vi "埃德1.vi"() -> ()   [LabVIEW 2017]
uses:
  <vilib>/vision/Pattern Matching.llb/IMAQ GM Match Report.ctl
panel:
  out "Matches (Geometric Matching 1)":T1[](array[typedef]) {"Correlation Score" format="%.2f"; "Target Template Curve Score" format="%.2f"; "Template Target Curve Score" format="%.2f"; "Bounding Box"."y" format="%.2f"; "Bounding Box"."x" format="%.2f"; "Position"."y" format="%.2f"; "Position"."x" format="%.2f"; "Score" format="%.2f"; "Scale" format="%.2f"; "Angle" format="%.2f"; "Occlusion %" format="%.2f"}
  out "路径":path
  out "数值":i32
  in  "毫秒计时值":u32
  out "Image":T2(plugin-control)
  out "All Files in Dir":path[](array[path]) caption="目录中的所有文件"
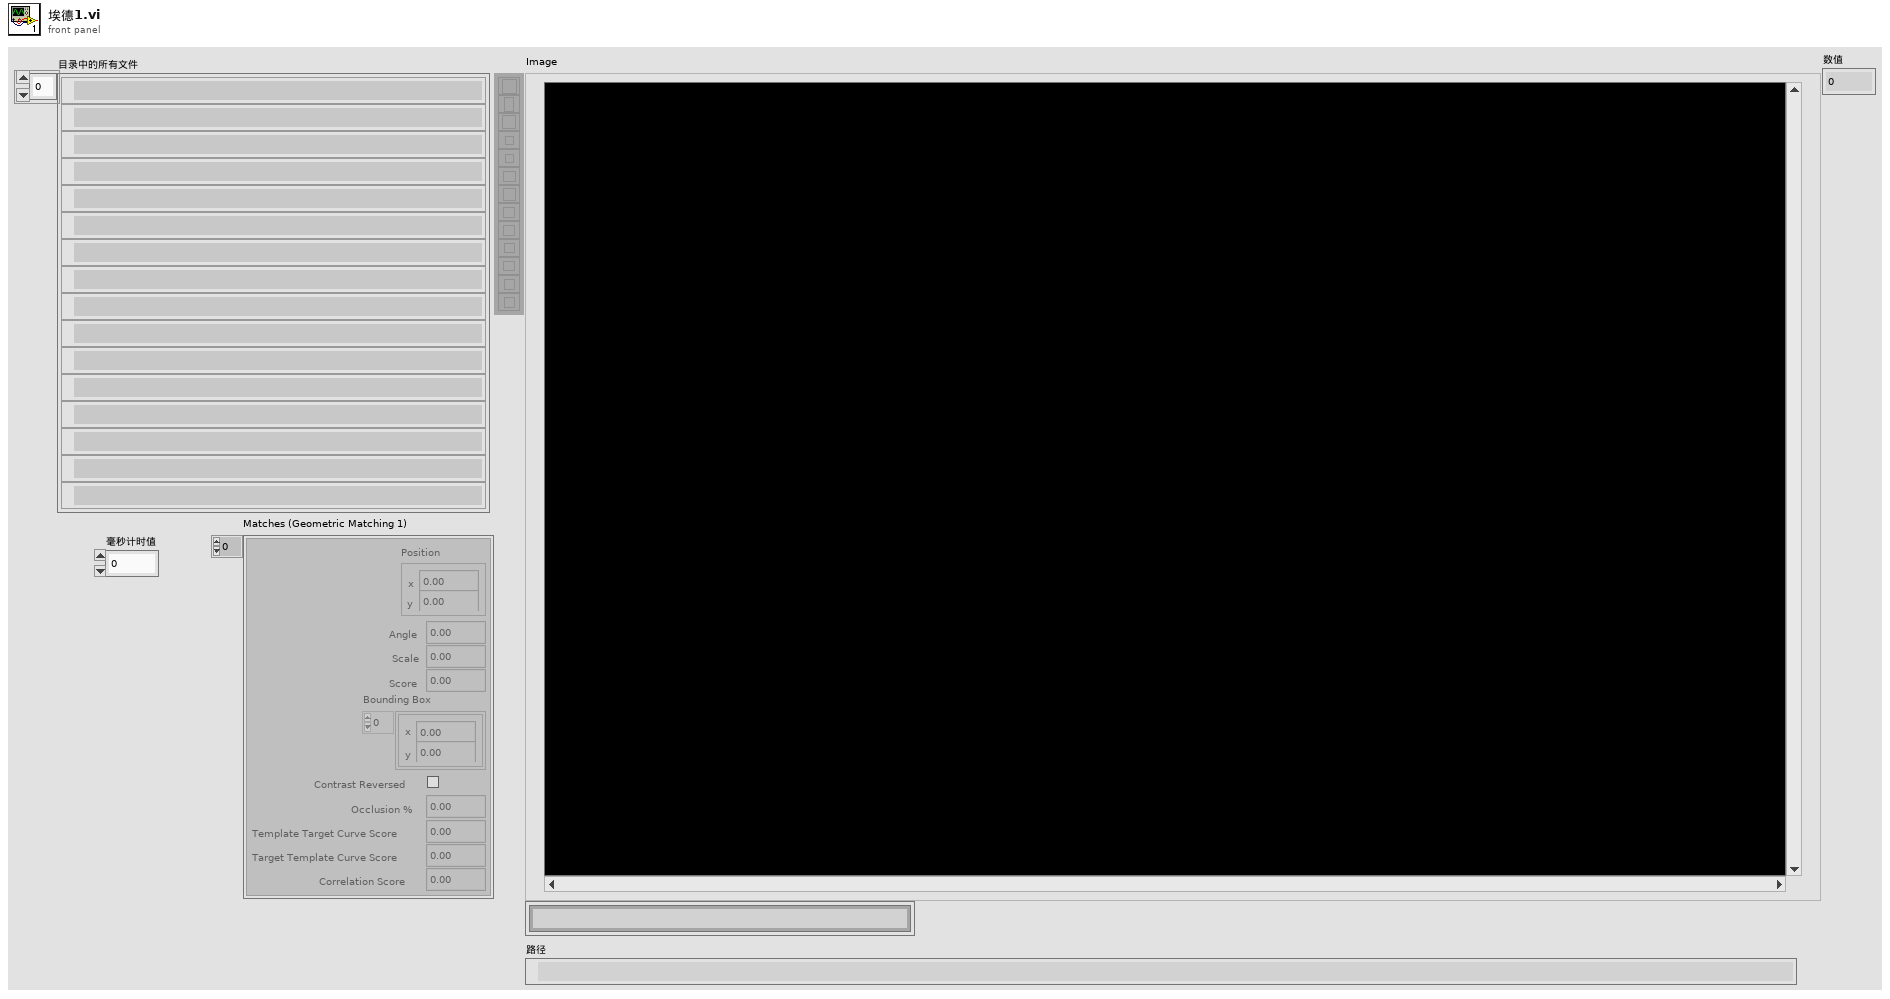
[diagram p1: front panel]
types:
  T1 = typedef "IMAQ GM Match Report.ctl" = cluster{"Position":cluster{"x":sgl, "y":sgl}, "Angle":sgl, "Scale":sgl, "Score":sgl, "Bounding Box":cluster{"x":sgl, "y":sgl}[], "Contrast Reversed":bool, "Occlusion %":sgl, "Template Target Curve Score":sgl, "Target Template Curve Score":sgl, "Correlation Score":sgl}
  T2 = typedef "IMAQ Image.ctl" = refnum<image>
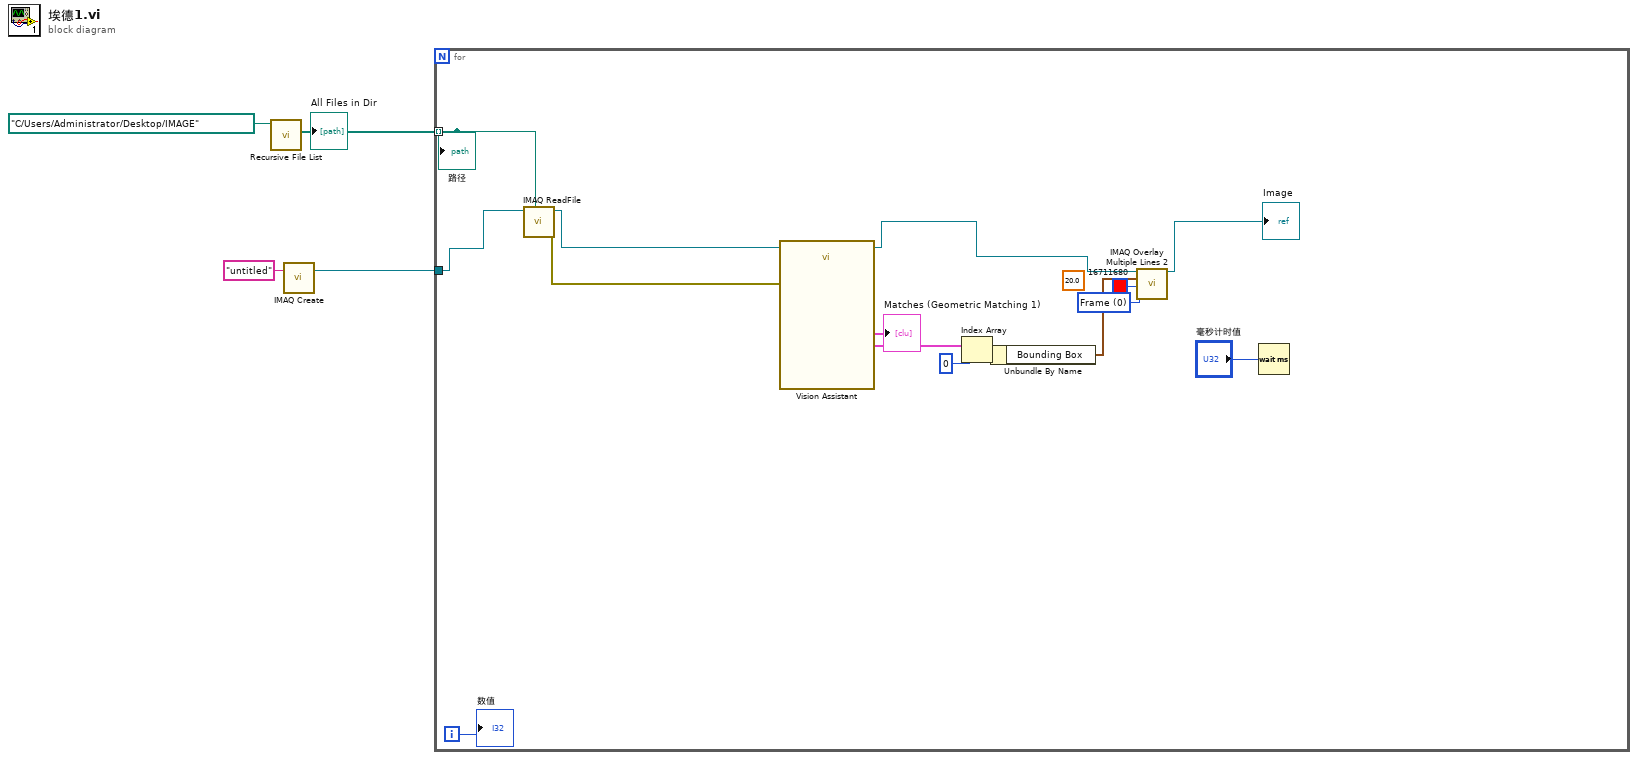
[diagram p0: block diagram]
diagram:
  n1 = call <vilib>:"Recursive File List.vi"("Folder Path"=path "C:/Users/Administrator/Desktop/IMAGE" ("path")) -> ("All Files in Dir"=w1:path[])  [unwired: 6 in, 4 out]
  "All Files in Dir" <- w1
  n2 = call "IMAQ Create"("Image Name"="untitled") -> ("New Image"=w2:T2)  [unwired: 4 in, 1 out]
  n3 = for {
    tunnel: w2 -> [w18]
    tunnel: w1 -> [w17] mode=indexing
    i -> [w13]
    w7 = u32 0 items=["Frame", "Fill"] ("Drawing Mode (Frame)")
    (unwired) 20.0 ("radius")
    n4 = call "IMAQ ReadFile"("File Path"=w17, "Image"=w18) -> ("error out"=w15:errorcluster, "Image Out"=w16:T2)  [unwired: 5 in, 3 out]
    n5 = call "Vision Assistant"("Image In"=w16, "error in"=w15) -> ("Image Out"=w9:T2, "Matches (Geometric Matching 1)"=w12:T1[])  [unwired: 21 in, 3 out]
    "Matches (Geometric Matching 1)" <- w12
    n6 = Index Array(array=w12, index=0 ("索引")) -> (element=w10:T1)
    n7 = Unbundle By Name(w10) -> ("Bounding Box"=w8:cluster{"x":sgl, "y":sgl}[])
    n8 = call "IMAQ Overlay Multiple Lines 2"("Image"=w9, "Line End Points"=w8, "Drawing Mode (Frame)"=w7, "Color"=u32 16711680) -> ("Image Out"=→"Image":T2)  [unwired: 10 in, 1 out]
    n9 = Wait (ms)(milliseconds to wait="毫秒计时值") -> ()  [unwired: 1 out]
    "数值" <- w13
    "路径" <- w17
  }
